vi "calcUkRefX00.vi"(8 "error in (no error)":errorcluster, 9 "dofIdx":i32[](array[numeric]), 10 "Qx Array":dbl[][](array[numeric]), 11 "OptCtrl in":refnum<class "OptCtrl.lvclass">) -> (0 "error out":errorcluster, 2 "uk Array":dbl[](array[numeric]), 3 "OptCtrl out":refnum<class "OptCtrl.lvclass">)   [LabVIEW 2016, in "OptCtrl.lvclass"]
doc: "Calculate uk by referencing to \"x00\". The offset will only trace the relative changes of offset without regarding the real value."
uses:
  OptCtrl.lvclass
  OptCtrl.lvclass/OptCtrl.ctl
  Utility/getSubArray1D.vi
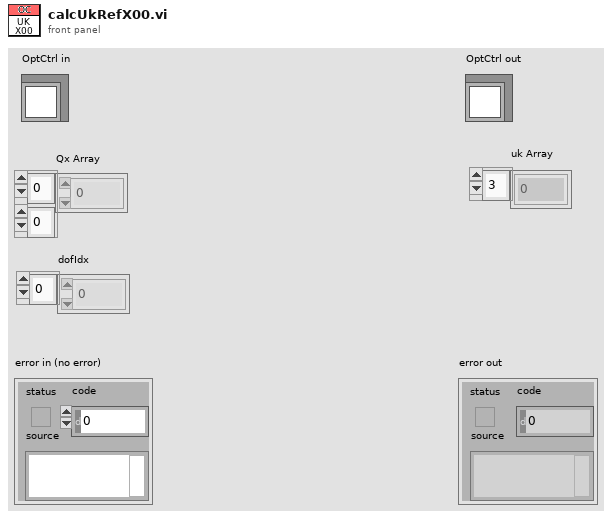
[diagram p1: front panel]
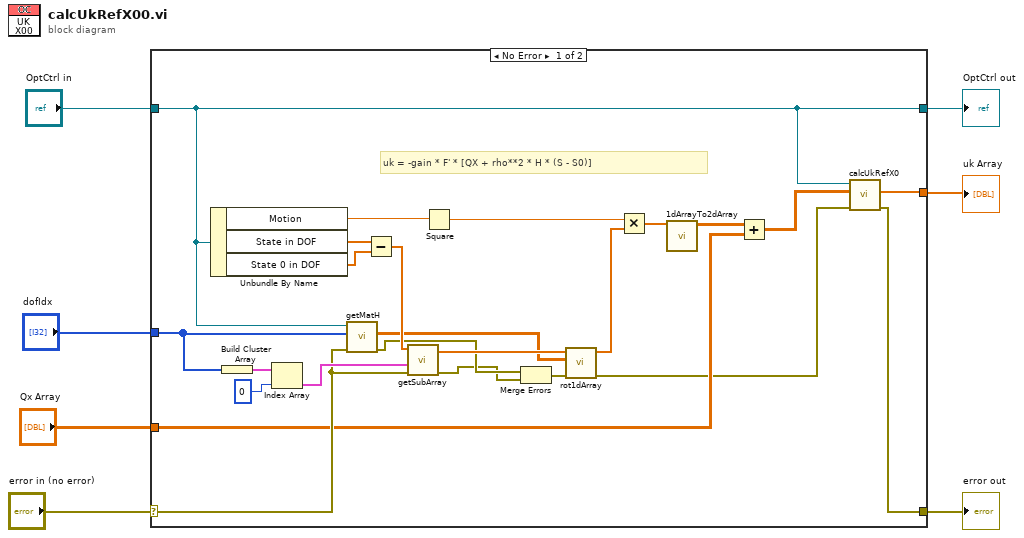
[diagram p0: block diagram]
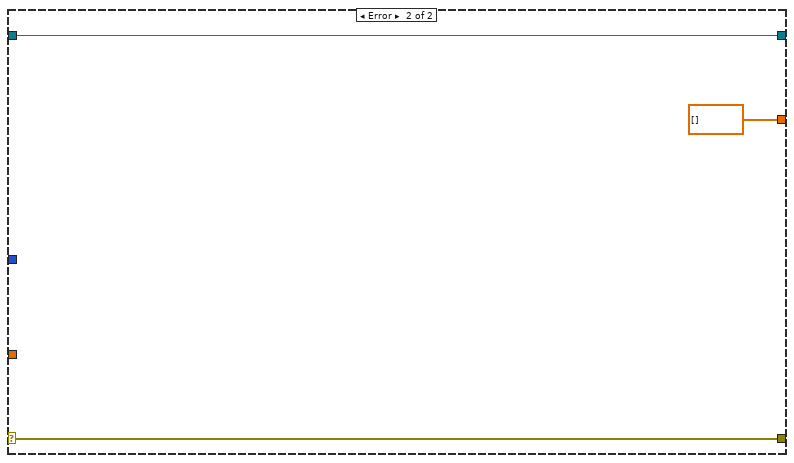
[diagram p2: hidden frame]
diagram:
  n1 = case shown="No Error" "error in (no error)" {
    selector: "error in (no error)" -> [w20 w34]
    tunnel: [w8 w34] -> w6
    tunnel: [w12 w33] -> w4
    tunnel: "OptCtrl in" -> [w12 w33]
    tunnel: "dofIdx" -> [w24 _]
    tunnel: "Qx Array" -> [w13 _]
    tunnel: [w11 dbl[] [] ("1D Array")] -> w1
    frame No Error {
      # "uk = -gain * F' * [QX + rho**2 * H * (S - S0)]"
      n2 = Unbundle By Name(w12) -> ("Motion"=w31:dbl, "State in DOF"=w29:dbl[], "State 0 in DOF"=w28:dbl[])
      n3 = Build Cluster Array(w24) -> (w27:cluster{"dofIdx":i32[]}[])
      n4 = Index Array(array=w27, index=0) -> (element=w25:cluster{"dofIdx":i32[]})
      n5 = call "getMatH.vi"("error in (no error)"=w20, "dofIdx"=w24, "OptCtrl in"=w12) -> ("error out"=w19:errorcluster, "Matrix H"=w21:dbl[][])  [unwired: 6 in, 1 out]
      n6 = Subtract(x=w29, y=w28) -> (x-y=w23:dbl[])
      n7 = call-poly "getSubArray.vi"("error in (no error)"=w20, "Index Array Cluster"=w25, "1D Array"=w23) -> ("error out"=w17:errorcluster, "Sub-Array"=w22:dbl[])  [unwired: 7 in]
      n8 = Square(x=w31) -> (x^2=w30:dbl)
      n9 = Merge Errors(w19, w17) -> (w18:errorcluster)
      n10 = call "rot1dArray.vi"("error in (no error)"=w18, "Rot Mat"=w21, "1D Array"=w22) -> ("error out"=w9:errorcluster, "Rotated 1D Array"=w16:dbl[])  [unwired: 7 in]
      n11 = Multiply(x=w30, y=w16) -> (x*y=w15:dbl[])
      n12 = call "1dArrayTo2dArray.vi"("1D Array"=w15) -> ("2D Array"=w14:dbl[][])  [unwired: 10 in]
      n13 = Add ("Add.vi")(x=w14, y=w13) -> (x+y=w10:dbl[][])
      n14 = call "calcUkRefX0.vi"("error in (no error)"=w9, "Qx Array"=w10, "OptCtrl in"=w12) -> ("error out"=w8:errorcluster, "uk Array"=w11:dbl[])  [unwired: 6 in, 1 out]
    }
    frame Error {
    }
  }
  "error out" <- w6
  "OptCtrl out" <- w4
  "uk Array" <- w1
